vi "test.vi"() -> ()   [LabVIEW 2016, in "TCP文件传输系统.lvlib"]
uses:
  <vilib>/Utility/sysdir.llb/System Directory Type.ctl
panel:
  out "文件传输的路径":path
  in  "字符串":string="平台数据传输系统.exe"
  in  "远程端口或服务名称":u16=11234
  out "本机网络地址":string="192.168.1.250"
  out "TCP发送全局簇":T1={"网络灯"=FALSE, "发送中"=TRUE, "已发送百分比"=0, "发送成功次数"=0.0}
  out "传输次数":dbl
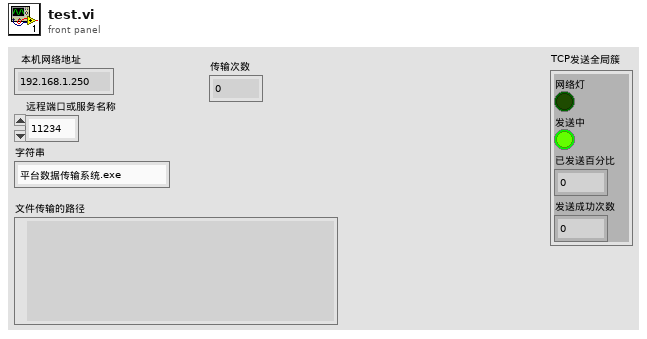
[diagram p1: front panel]
types:
  T1 = cluster{"网络灯":bool, "发送中":bool, "已发送百分比":u8, "发送成功次数":dbl}
  T2 = typedef "System Directory Type.ctl" = i32
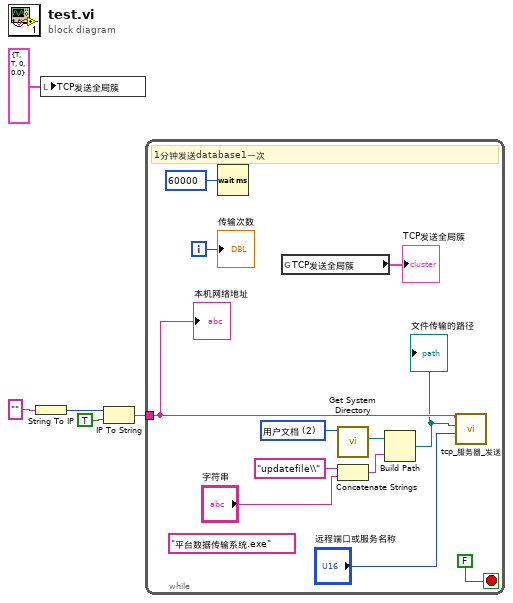
[diagram p0: block diagram]
diagram:
  n1 = String To IP(1:"" ("名称")) -> (0:w4:u32)
  n2 = local write "TCP发送全局簇"(T1 {"网络灯"=TRUE, "发送中"=TRUE, "已发送百分比"=0, "发送成功次数"=0.0} ("TCP发送全局簇")) -> ()
  n3 = IP To String(1:TRUE ("句点符号？(F)"), 2:w4) -> (0:w1:string)
  n4 = while {
    tunnel: w1 -> [w8]
    i -> [w11]
    stop <- FALSE stop-if-true
    (unwired) "平台数据传输系统.exe" ("字符串")
    w15 = T2 2 items=["用户目录"=0, "用户桌面"=1, "用户文档"=2, "用户应用程序数据"=3, "用户设置"=4, "用户临时目录"=5, "公共文档"=6, "公共应用程序数据"=7, "公共设置"=8, "公共缓存"=13, "系统核心库"=9, "系统安装库"=10, "应用程序文件"=11, "启动盘根目录"=12] ("system directory type")
    # "1分钟发送database1一次"
    n5 = Wait (ms)(milliseconds to wait=u32 60000 ("等待时间（毫秒）")) -> ()  [unwired: 1 out]
    n6 = global read "全局变量1.vi" "TCP发送全局簇"() -> (→"TCP发送全局簇":T1)
    n7 = call <vilib>:"Get System Directory.vi"("system directory type"=w15) -> ("system directory"=w14:path)  [unwired: 10 in]
    n8 = Concatenate Strings("updatefile\\" ("condition"), "字符串") -> (w12:string)
    n9 = Build Path(base path=w14, name or relative path=w12) -> (appended path=w7:path)
    "文件传输的路径" <- w7
    n10 = call "tcp_服务器_发送.vi"("远程端口或服务名称"="远程端口或服务名称", "原文件路径（使用对话框）"=w7, "服务器网络地址"=w8) -> ()  [unwired: 9 in]
    "传输次数" <- w11
    "本机网络地址" <- w8
  }
